vi "Add From Spreadsheet.vi"(7 "file path (use dialog)":path, 8 "error in (no error)":errorcluster, 11 "Item Ref":T1 format="%.0x") -> (0 "error out":errorcluster)   [LabVIEW 2020, in "RefMem DMA System Explorer.lvlib"]
uses:
  RefMem DMA System Explorer.lvlib
  <vilib>/NI VeriStand/Custom Device API/Custom Device Item Ref.ctl
  <vilib>/NI VeriStand/Custom Device API/Custom Device Channel.ctl
  <vilib>/NI VeriStand/Custom Device API/Custom Device Channel Type.ctl
  controls/Data Channel Type.ctl
  Shared/Constants.vi
  <vilib>/NI VeriStand/Custom Device API/Set Item Property (U16).vi
  <vilib>/NI VeriStand/Custom Device API/Set Item Property (U32).vi
  Shared/RefMem DMA Shared.lvlib
  <vilib>/NI VeriStand/Custom Device API/Custom Device API.lvlib
panel:
  out "array w/ subset deleted":string[][](array[string])
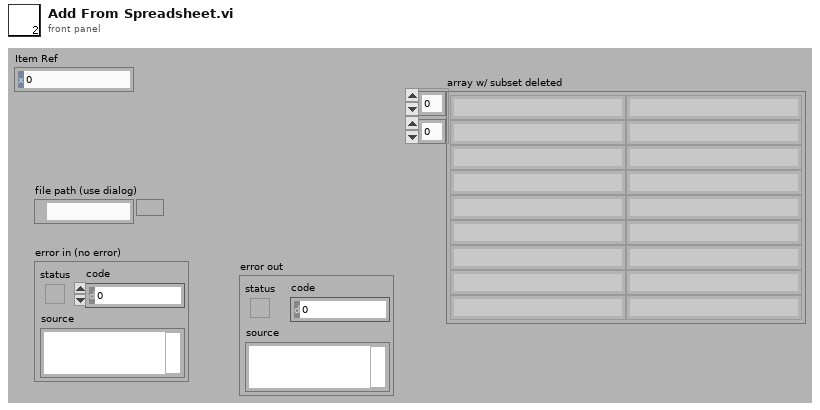
[diagram p1: front panel]
types:
  T1 = typedef "Custom Device API.lvlib/Custom Device Item Ref.ctl" = u64
  T2 = typedef "Custom Device API.lvlib/Custom Device Channel.ctl" = cluster{"Type":T3, "Units":string, "Default Value":dbl, "Faultable":bool, "Scalable":bool}
  T3 = typedef "Custom Device API.lvlib/Custom Device Channel Type.ctl" = enum16{"Input", "Output"}
  T4 = typedef "RefMem DMA System Explorer.lvlib/Data Channel Type.ctl" = enum16{"Read", "Write"}
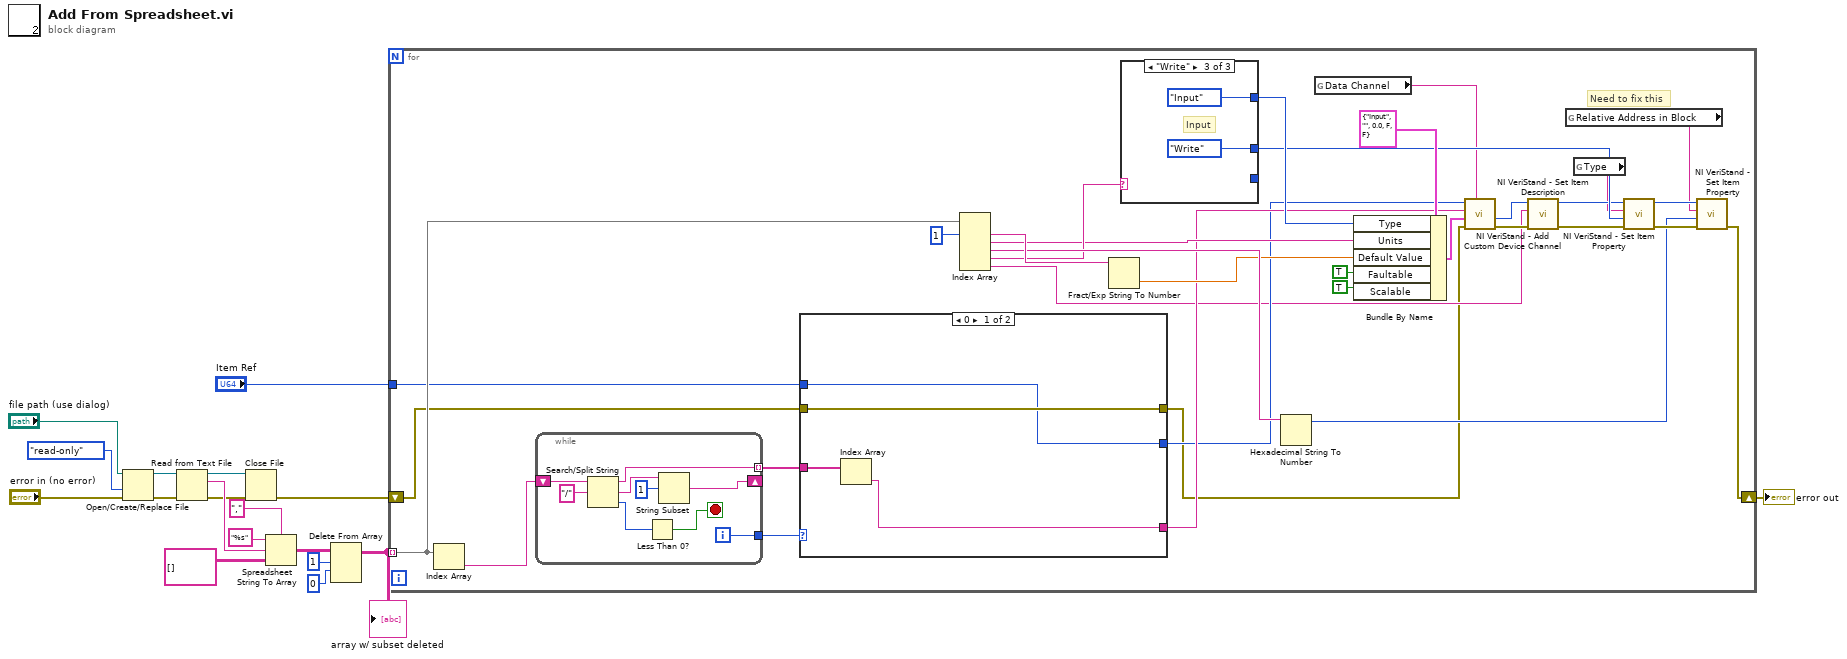
[diagram p0: block diagram]
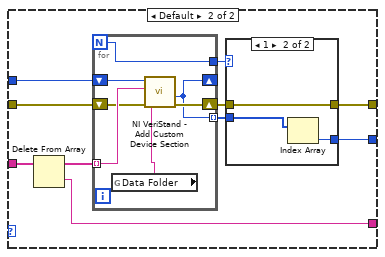
[diagram p2: hidden frame]
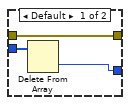
[diagram p3: hidden frame]
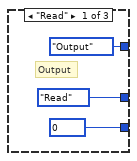
[diagram p4: hidden frame]
diagram:
  n1 = Open/Create/Replace File(file path (use dialog)="file path (use dialog)", error in="error in (no error)", access (0:read/write)=enum16{"read/write", "read-only", "write-only"}."read-only") -> (refnum out=w8:refnum<file>, error out=w7:errorcluster)  [unwired: 3 in, 1 out]
  n2 = Read from Text File(file (use dialog)=w8, error in=w7) -> (refnum out=w9:refnum<file>, text=w12:string, error out=w10:errorcluster)  [unwired: 2 in, 1 out]
  n3 = Close File(refnum=w9, error in=w10) -> (error out=w18:errorcluster)  [unwired: 1 out]
  n4 = Spreadsheet String To Array(delimiter (Tab)=",", format string="%s", spreadsheet string=w12, array type (2D Dbl)=string[][] []) -> (array=w14:string[][])
  n5 = Delete From Array(array=w14, length=1, index (row)=0) -> (array with subset deleted=w17:string[][])  [unwired: 1 in, 1 out]
  "array w/ subset deleted" <- w17
  n6 = for {
    tunnel: w17 -> [w51] mode=indexing
    shift-right: [w19] -> w2
    shift-left: w18 -> [w24]
    tunnel: "Item Ref" -> [w31]
    # "Need to fix this"
    n7 = Index Array(array=w51) -> (element=w33:string)  [unwired: 1 in]
    n8 = while {
      tunnel: [w83] -> w34 mode=indexing
      shift-right: [w81] -> _
      shift-left: w33 -> [w87]
      tunnel: [w79] -> w35
      i -> [w79]
      stop <- w84 stop-if-true
      n9 = Search/Split String(string=w87, search string/char (-)="/") -> (substring before match=w83:string, match + rest of string=w82:string, offset of match=w85:i32)  [unwired: 1 in]
      n10 = Less Than 0?(x=w85) -> (x < 0?=w84:bool)
      n11 = String Subset(string=w82, offset (0)=1) -> (substring=w81:string)  [unwired: 1 in]
    }
    n12 = case shown="0" w35 {
      tunnel: [w55 w59] -> w20
      tunnel: w24 -> [w55 w64]
      tunnel: w34 -> [w54 w65]
      tunnel: w31 -> [w52 w57]
      tunnel: [w53 w58] -> w32
      tunnel: [w52 w56] -> w30
      frame 0 {
        n13 = Index Array(array=w54) -> (element=w53:string)  [unwired: 1 in]
      }
      frame Default {
        n14 = Delete From Array(array=w65) -> (deleted portion=w58:string, array with subset deleted=w63:string[])  [unwired: 2 in]
        n15 = for {
          N -> [w78]
          shift-right: [w74] -> w60
          shift-left: w64 -> [w75]
          shift-right: [w72] -> _
          shift-left: w57 -> [w73]
          tunnel: w63 -> [w77] mode=indexing
          tunnel: [w72] -> w61 mode=indexing
          tunnel: [w78] -> w62
          n16 = global read "Constants.vi" "Data Folder"() -> (w76:string)
          n17 = call <vilib>:"NI VeriStand - Add Custom Device Section.vi"("GUID (Default Section)"=w76, "error in (no error)"=w75, "Section Name"=w77, "Parent Ref in"=w73) -> ("error out"=w74:errorcluster, "Section Ptr"=w72:T1)  [unwired: 4 in, 2 out]
        }
        n18 = case shown="1" w62 {
          tunnel: w61 -> [w68 w71]
          tunnel: [w67 w70] -> w56
          tunnel: w60 -> [w66 w69]
          tunnel: [w66 w69] -> w59
          frame Default {
            n19 = Delete From Array(array=w68) -> (deleted portion=w67:T1)  [unwired: 2 in, 1 out]
          }
          frame 1 {
            n20 = Index Array(array=w71) -> (element=w70:T1)  [unwired: 1 in]
          }
        }
      }
    }
    n21 = Index Array(array=w51, index #1=1 ("index")) -> (element #1=w49:string, element #2=w44:string, element #3=w48:string, element #4=w47:string, element #5=w26:string)  [unwired: 4 in]
    n22 = Fract/Exp String To Number(string=w49) -> (number=w43:dbl)  [unwired: 3 in, 1 out]
    n23 = case shown="\"Write\"" w47 {
      tunnel: [Data_Channel_Type."Read" ("Type") _ Data_Channel_Type."Write" ("Type")] -> w39
      tunnel: [u32 0 ("BitFields") _ _] -> _
      tunnel: [Custom_Device_Channel_Type."Output" ("Type") _ Custom_Device_Channel_Type."Input" ("Type")] -> w40
      frame "Read" {
        # "Output"
      }
      frame Default {
      }
      frame "Write" {
        # "Input"
      }
    }
    n24 = Hexadecimal String To Number(string=w48) -> (number=w36:u32)  [unwired: 2 in, 1 out]
    n25 = global read "Constants.vi" "Data Channel"() -> (w21:string)
    n26 = Bundle By Name(cluster=T2 {"Type"=enum."Input", "Units"="", "Default Value"=0.0, "Faultable"=FALSE, "Scalable"=FALSE} ("Channel"), "Type"=w40, "Units"=w44, "Default Value"=w43, "Faultable"=TRUE, "Scalable"=TRUE) -> (w45:T2)
    n27 = call <vilib>:"NI VeriStand - Add Custom Device Channel.vi"("GUID (Default Channel)"=w21, "error in (no error)"=w20, "Channel"=w45, "Channel Name"=w32, "Parent Ref in"=w30) -> ("error out"=w29:errorcluster, "Channel Ref"=w25:T1)  [unwired: 3 in, 2 out]
    n28 = call <vilib>:"NI VeriStand - Set Item Description.vi"("error in (no error)"=w29, "Description"=w26, "Item Ref in"=w25) -> ("error out"=w28:errorcluster, "Item Ref out"=w27:T1)  [unwired: 6 in, 1 out]
    n29 = global read "Constants.vi" "Relative Address in Block"() -> (w23:string)
    n30 = global read "Constants.vi" "Type"() -> (w22:string)
    n31 = call-poly <vilib>:"NI VeriStand - Set Item Property.vi"("error in (no error)"=w28, "Value"=w39, "Property Name"=w22, "Item Ref in"=w27) -> ("error out"=w37:errorcluster, "Item Ref out"=w38:T1)  [unwired: 5 in, 1 out]
    n32 = call-poly <vilib>:"NI VeriStand - Set Item Property.vi"("error in (no error)"=w37, "Value"=w36, "Property Name"=w23, "Item Ref in"=w38) -> ("error out"=w19:errorcluster)  [unwired: 5 in, 2 out]
  }
  "error out" <- w2
